vi "ui.vi"() -> ()   [LabVIEW 2018]
uses:
  <userlib>/ROS for LabVIEW Software/ROS/Code/Console/Servers/ServerSubs/TopicDef.ctl
  <userlib>/ROS for LabVIEW Software/ROS/Code/SubVIs/_ROSDirection.ctl
  <userlib>/ROS for LabVIEW Software/ROS/Code/_ROSDefinition.vi
  <userlib>/ROS for LabVIEW Software/ROS/MessageBuilding/std_msgs/subs/boolScalar.vi
  <userlib>/ROS for LabVIEW Software/ROS/MessageBuilding/std_msgs/subs/u32Scalar.vi
panel:
  in  "Tab Control":enum32{"Control & Monitor", "State", "Setting"}(tab)
  in  "roscore":bool
  in  "mt4n":bool
  in  "xclock":bool
  in  "AGV Stop":bool
  in  "AGV CCW":bool
  in  "AGV CW":bool
  in  "AGV Left":bool
  in  "ARV Right":bool
  in  "AGV Rear":bool
  in  "AGV Front":bool
  out "batteryState sub":T1
  out "stop":bool
  in  "Mode":T2(ring)
  out "event(ms)":u32
  in  "rqt":bool
  out "Init Chk(s)":dbl
  in  "Init Time(s)":dbl=3.0
  out "labview_ui retry count":i32
  out "mt4n retry count":i32
  out "xclock(std out)":string
  out "xclock(std err)":string
  out "xclock(ret)":i32
  out "xclock(err)":errorcluster
  out "mt4n(std out)":string
  out "mt4n(std err)":string
  out "mt4n(ret)":i32
  out "mt4n(err)":errorcluster
  out "roscore(std out)":string
  out "roscore(std err)":string
  out "roscore(ret)":i32
  out "roscore(err)":errorcluster
  out "rqt(err)":errorcluster
  out "rqt(ret)":i32
  out "rqt(std err)":string
  out "rqt(std out)":string
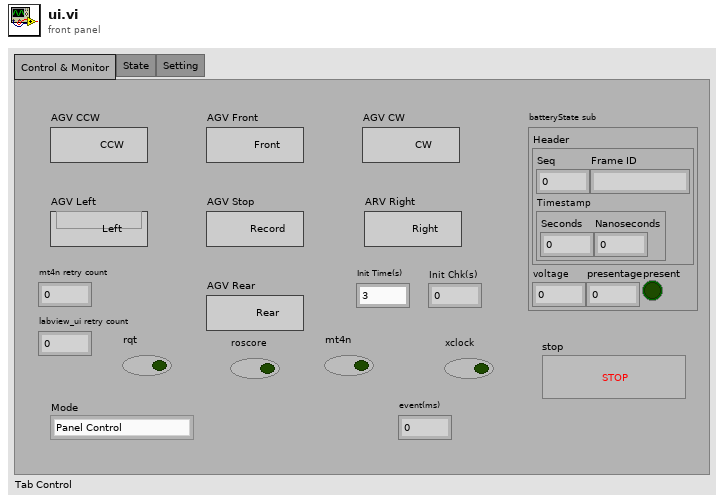
[diagram p1: front panel]
types:
  T1 = cluster{"Header":cluster{"Seq":u32, "Frame ID":string, "Timestamp":cluster{"Seconds":i32, "Nanoseconds":i32}}, "voltage":sgl, "presentage":sgl, "present":bool}
  T2 = enum16{"Panel Control", "Joystick", "Jeong-Hwan Kwak", "Sang Mun Lee"}
  T3 = enum32{"invalid app kind", "Development System", "Run Time System", "Student Edition", "Embedded LabVIEW", "Evaluation", "Custom"}
  T4 = typedef "TopicDef.ctl" = cluster{"Topic":string, "Type":string, "Action":T5, "Update (ms)":u16, "queue size":u16}
  T5 = typedef "_ROSDirection.ctl" = enum16{"Node", "Publisher", "Subscriber", "ServiceClient", "ServiceProvider"}
  T6 = typedef "_ROSControl.ctl" = cluster{"topic port":u16, "Node":string, "topic":string, "type":string, "node port":u16, "error ":errorcluster, "Direction":T5, "Update (ms)":u16, "FIFO size":u16}
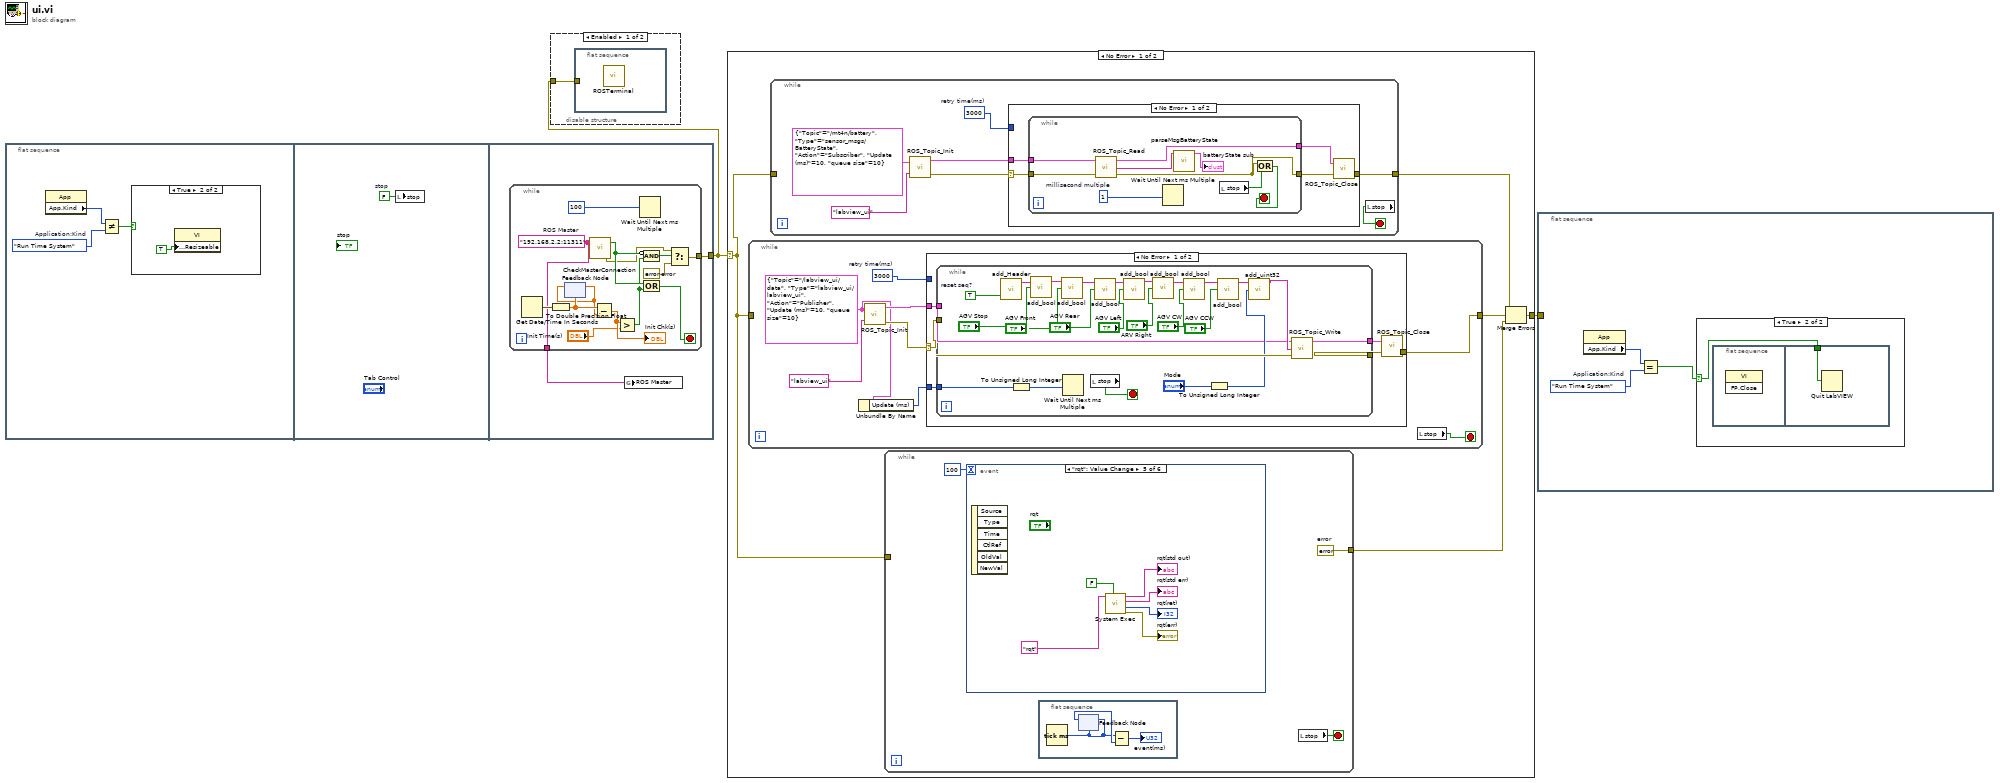
[diagram p0: block diagram]
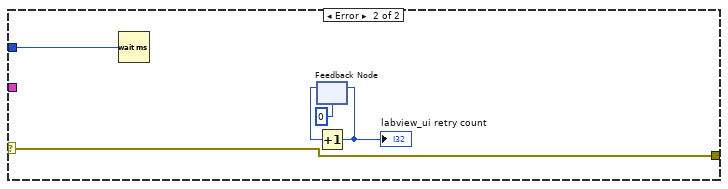
[diagram p3: hidden frame]
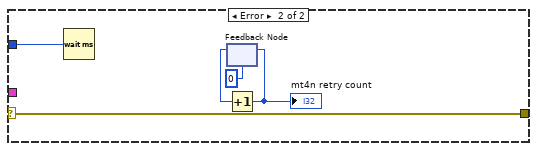
[diagram p4: hidden frame]
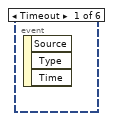
[diagram p5: hidden frame]
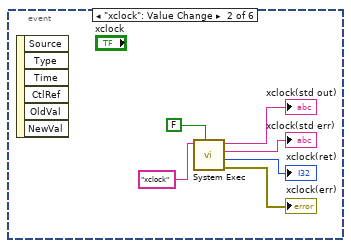
[diagram p6: hidden frame]
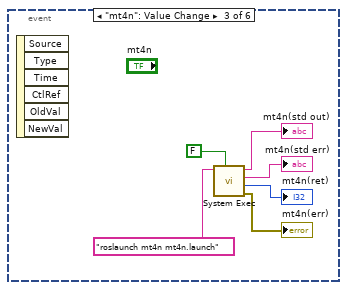
[diagram p7: hidden frame]
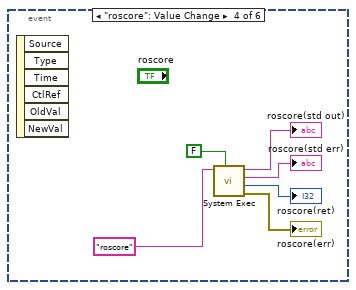
[diagram p8: hidden frame]
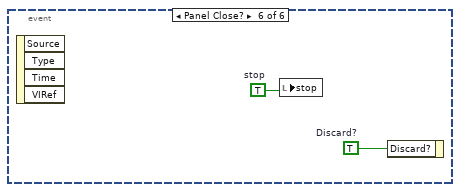
[diagram p9: hidden frame]
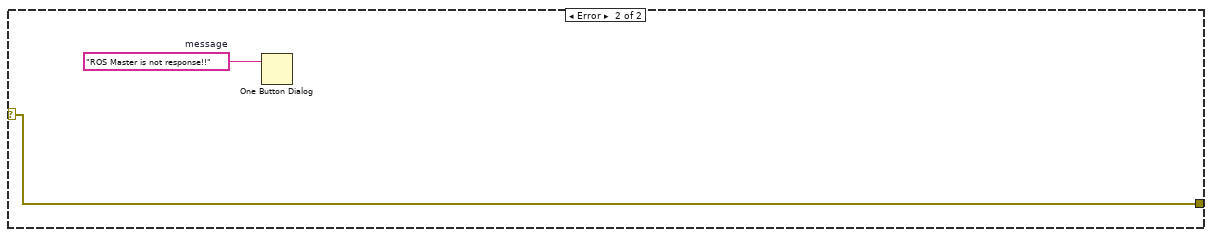
[diagram p10: hidden frame]
diagram:
  n1 = flat-sequence {
    tunnel: [w9] -> w1
    frame #0 {
      w3 = T3."Run Time System"  # Application:Kind
      n2 = property class="App"() -> ("App.Kind"=w4:T3)  [unwired: 2 in, 2 out]
      n3 = Not Equal?(x=w4, y=w3) -> (x != y?=w5:bool)
      n4 = case shown="True" w5 {
        frame False {
        }
        frame True {
          n5 = property class="VI"("Front Panel.Resizeable"=TRUE) -> ()  [unwired: 2 in, 2 out]
        }
      }
    }
    frame #1 {
      w7 = FALSE  # stop
      n6 = local write "stop"(w7) -> ()
    }
    frame #2 {
      n7 = while {
        tunnel: [w13] -> w9
        tunnel: [w10] -> w8
        stop <- w18 stop-if-true
        w12 = errorcluster {"status"=FALSE, "code"=0, "source"=""}  # error
        w10 = "192.168.2.2:11311"  # ROS Master
        n8 = Get Date/Time In Seconds() -> (seconds since 1Jan1904=w23:timestamp)
        n9 = To Double Precision Float(number=w23) -> (double precision float=w22:dbl)
        n10 = feedback #1(w22) -> (w21:dbl)
        n11 = feedback-in #1(w21) -> ()
        n12 = call <userlib>:"CheckMasterConnection.vi"("Master IP"=w10) -> ("error out"=w11:errorcluster, "Master There?"=w16:bool)  [unwired: 1 in]
        n13 = Subtract(x=w22, y=w21) -> (x-y=w20:dbl)
        "Init Chk(s)" <- w20
        n14 = Greater?(x=w20, y="Init Time(s)") -> (0:w15:bool)
        n15 = Wait Until Next ms Multiple(millisecond multiple=u32 100) -> ()  [unwired: 1 out]
        n16 = Compound Arithmetic op=AND(invert w16, w15) -> (w14:bool)
        n17 = Compound Arithmetic op=OR(w16, w15) -> (w18:bool)
        n18 = Select(t=w11, s=w14, f=w12) -> (s? t:f=w13:errorcluster)
      }
      n19 = global write "_ROSDefinition.vi" "ROS Master"(w8) -> ()
    }
  }
  n20 = disable-structure shown="Enabled" {
    disable-tunnel: w1 -> [w24 _]
    frame Enabled {
      n21 = flat-sequence {
        tunnel: w24 -> [_]
        frame #0 {
          n22 = call <userlib>:"ROSTerminal.vi"() -> ()  [unwired: 2 in]
        }
      }
    }
    frame Disabled {
    }
  }
  n23 = case shown="No Error" w1 {
    selector: w1 -> [w25 w134]
    tunnel: [w26 w134] -> w2
    frame No Error {
      n24 = while {
        tunnel: w25 -> [_]
        tunnel: [w36] -> w28
        stop <- w34 stop-if-true
        w32 = u32 3000  # retry time(ms)
        w31 = T4 {"Topic"="/labview_ui/data", "Type"="labview_ui/labview_ui", "Action"=enum."Publisher", "Update (ms)"=10, "queue size"=10} ("Definitions")
        n25 = Unbundle By Name(w31) -> ("Update (ms)"=w30:u16)
        n26 = call <userlib>:"ROS_Topic_Init.vi"("Definitions"=w31, "node"="labview_ui") -> ("ROS out"=w37:T6, "error out"=w33:errorcluster)  [unwired: 1 in]
        n27 = case shown="No Error" w33 {
          selector: w33 -> [w39 w70]
          tunnel: w37 -> [w41 _]
          tunnel: [w40 w70] -> w36
          tunnel: w32 -> [_ w74]
          tunnel: w30 -> [w38 _]
          frame No Error {
            n28 = while {
              tunnel: w41 -> [w46]
              tunnel: w39 -> [w69]
              tunnel: [w68] -> w42
              tunnel: [w67] -> w43
              tunnel: w38 -> [w45]
              stop <- w66 stop-if-true
              w65 = TRUE  # reset seq?
              n29 = call <userlib>:"add_Header.vi"("reset seq?"=w65) -> ("msg out"=w56:string)  [unwired: 4 in]
              n30 = To Unsigned Long Integer(number=w45) -> (unsigned 32bit integer=w44:u32)
              n31 = call-poly <userlib>:"add_bool.vi"("Boolean"="AGV Stop", "msg in"=w56) -> ("msg out"=w55:string)  [unwired: 3 in]
              n32 = call-poly <userlib>:"add_bool.vi"("Boolean"="AGV Front", "msg in"=w55) -> ("msg out"=w54:string)  [unwired: 3 in]
              n33 = Wait Until Next ms Multiple(millisecond multiple=w44) -> ()  [unwired: 1 out]
              n34 = local read "stop"() -> (w66:bool)
              n35 = call-poly <userlib>:"add_bool.vi"("Boolean"="AGV Rear", "msg in"=w54) -> ("msg out"=w53:string)  [unwired: 3 in]
              n36 = call-poly <userlib>:"add_bool.vi"("Boolean"="AGV Left", "msg in"=w53) -> ("msg out"=w50:string)  [unwired: 3 in]
              n37 = call-poly <userlib>:"add_bool.vi"("Boolean"="ARV Right", "msg in"=w50) -> ("msg out"=w51:string)  [unwired: 3 in]
              n38 = call-poly <userlib>:"add_bool.vi"("Boolean"="AGV CW", "msg in"=w51) -> ("msg out"=w52:string)  [unwired: 3 in]
              n39 = To Unsigned Long Integer(number="Mode") -> (unsigned 32bit integer=w47:u32)
              n40 = call-poly <userlib>:"add_bool.vi"("Boolean"="AGV CCW", "msg in"=w52) -> ("msg out"=w49:string)  [unwired: 3 in]
              n41 = call-poly <userlib>:"add_uint32.vi"("Numeric"=w47, "msg in"=w49) -> ("msg out"=w57:string)  [unwired: 3 in]
              n42 = call <userlib>:"ROS_Topic_Write.vi"("error in (no error)"=w69, "Msg in"=w57, "ROS in"=w46) -> ("error out"=w67:errorcluster, "ROS out"=w68:T6)  [unwired: 1 in]
            }
            n43 = call <userlib>:"ROS_Topic_Close.vi"("error in"=w43, "ROS in"=w42) -> ("error out"=w40:errorcluster)  [unwired: 2 in]
          }
          frame Error {
            n44 = Wait (ms)(milliseconds to wait=w74) -> ()  [unwired: 1 out]
            n45 = feedback #2(0) -> (w73:i32)
            n46 = Increment(x=w73) -> (x+1=w72:i32)
            "labview_ui retry count" <- w72
            n47 = feedback-in #2(w72) -> ()
          }
        }
        n48 = local read "stop"() -> (w34:bool)
      }
      n49 = while {
        tunnel: w25 -> [_]
        tunnel: [w80] -> w29
        stop <- w77 stop-if-true
        w75 = u32 3000  # retry time(ms)
        n50 = call <userlib>:"ROS_Topic_Init.vi"("Definitions"=T4 {"Topic"="/mt4n/battery", "Type"="sensor_msgs/BatteryState", "Action"=enum."Subscriber", "Update (ms)"=10, "queue size"=10}, "node"="labview_ui") -> ("ROS out"=w81:T6, "error out"=w76:errorcluster)  [unwired: 1 in]
        n51 = case shown="No Error" w76 {
          selector: w76 -> [w82 w97]
          tunnel: w81 -> [w86 _]
          tunnel: [w85 w97] -> w80
          tunnel: w75 -> [_ w96]
          frame No Error {
            n52 = while {
              tunnel: w86 -> [w87]
              tunnel: w82 -> [w95]
              tunnel: [w94] -> w83
              tunnel: [w88] -> w84
              stop <- w89 stop-if-true
              w91 = u32 1  # millisecond multiple
              n53 = call <userlib>:"ROS_Topic_Read.vi"("error in (no error)"=w95, "ROS in"=w87) -> ("error out"=w88:errorcluster, "Reply"=w93:string, "ROS out"=w94:T6)  [unwired: 1 in]
              n54 = Wait Until Next ms Multiple(millisecond multiple=w91) -> ()  [unwired: 1 out]
              n55 = call "parseMsgBatteryState.vi"("msg"=w93) -> ("batteryState"=→"batteryState sub":T1)  [unwired: 9 in, 1 out]
              n56 = local read "stop"() -> (w90:bool)
              n57 = Compound Arithmetic op=OR(w88, w90) -> (w89:bool)
            }
            n58 = call <userlib>:"ROS_Topic_Close.vi"("error in"=w84, "ROS in"=w83) -> ("error out"=w85:errorcluster)  [unwired: 2 in]
          }
          frame Error {
            n59 = Wait (ms)(milliseconds to wait=w96) -> ()  [unwired: 1 out]
            n60 = feedback #3(0) -> (w98:i32)
            n61 = Increment(x=w98) -> (x+1=w99:i32)
            "mt4n retry count" <- w99
            n62 = feedback-in #3(w99) -> ()
          }
        }
        n63 = local read "stop"() -> (w77:bool)
      }
      n64 = while {
        tunnel: w25 -> [_]
        tunnel: [w101] -> w27
        stop <- w103 stop-if-true
        w101 = errorcluster {"status"=FALSE, "code"=0, "source"=""}  # error
        n65 = event shown="[4] \"rqt\": Value Change" {
          selector: _ -> [_ _ _ _ _ _]
          dyn-events: _ -> [_ _ _ _ _ _]
          timeout: 100 -> [_ _ _ _ _ _]
          event Timeout {
            n66 = event-data() -> ()  [unwired: 1 in, 3 out]
          }
          event "xclock": Value Change {
            n67 = event-data() -> ()  [unwired: 1 in, 6 out]
            n68 = call <vilib>:"System Exec.vi"("wait until completion? (T)"=FALSE, "command line"="xclock") -> ("error out"=→"xclock(err)":errorcluster, "return code"=→"xclock(ret)":i32, "standard error"=→"xclock(std err)":string, "standard output"=→"xclock(std out)":string)  [unwired: 6 in]
          }
          event "mt4n": Value Change {
            n69 = event-data() -> ()  [unwired: 1 in, 6 out]
            n70 = call <vilib>:"System Exec.vi"("wait until completion? (T)"=FALSE, "command line"="roslaunch mt4n mt4n.launch") -> ("error out"=→"mt4n(err)":errorcluster, "return code"=→"mt4n(ret)":i32, "standard error"=→"mt4n(std err)":string, "standard output"=→"mt4n(std out)":string)  [unwired: 6 in]
          }
          event "roscore": Value Change {
            n71 = event-data() -> ()  [unwired: 1 in, 6 out]
            n72 = call <vilib>:"System Exec.vi"("wait until completion? (T)"=FALSE, "command line"="roscore") -> ("error out"=→"roscore(err)":errorcluster, "return code"=→"roscore(ret)":i32, "standard error"=→"roscore(std err)":string, "standard output"=→"roscore(std out)":string)  [unwired: 6 in]
          }
          event "rqt": Value Change {
            n73 = event-data() -> ()  [unwired: 1 in, 6 out]
            n74 = call <vilib>:"System Exec.vi"("wait until completion? (T)"=FALSE, "command line"="rqt") -> ("error out"=→"rqt(err)":errorcluster, "return code"=→"rqt(ret)":i32, "standard error"=→"rqt(std err)":string, "standard output"=→"rqt(std out)":string)  [unwired: 6 in]
          }
          event Panel Close? {
            w131 = TRUE  # Discard?
            w132 = TRUE  # stop
            n75 = event-data() -> ()  [unwired: 1 in, 4 out]
            n76 = local write "stop"(w132) -> ()
            n77 = event-data("Discard?"=w131) -> ()  [unwired: 1 in, 1 out]
          }
        }
        n78 = flat-sequence {
          frame #0 {
            n79 = Tick Count (ms)() -> (millisecond timer value=w105:u32)
            n80 = feedback #4(w105) -> (w106:u32)
            n81 = feedback-in #4(w105) -> ()
            n82 = Subtract(x=w105, y=w106) -> (x-y=→"event(ms)":u32)
          }
        }
        n83 = local read "stop"() -> (w103:bool)
      }
      n84 = Merge Errors(w29, w28, w27) -> (w26:errorcluster)
    }
    frame Error {
      w133 = "ROS Master is not response!!"  # message
      n85 = One Button Dialog(message=w133) -> ()  [unwired: 1 in, 1 out]
    }
  }
  n86 = flat-sequence {
    tunnel: w2 -> [_]
    frame #0 {
      w136 = T3."Run Time System"  # Application:Kind
      n87 = property class="App"() -> ("App.Kind"=w137:T3)  [unwired: 2 in, 2 out]
      n88 = Equal?(x=w137, y=w136) -> (x = y?=w135:bool)
      n89 = case shown="True" w135 {
        selector: w135 -> [_ w138]
        frame False {
        }
        frame True {
          n90 = flat-sequence {
            tunnel: w138 -> [w139]
            frame #0 {
              n91 = invoke class="VI" method="FP.Close"() -> ()  [unwired: 3 in, 3 out]
            }
            frame #1 {
              n92 = Quit LabVIEW(quit? (T)=w139) -> ()
            }
          }
        }
      }
    }
  }
